vi "Initialize.vi"(8 "error in (no error)":errorcluster, 9 "Reset (True)":bool=TRUE, 10 "ID Query (True)":bool=TRUE, 11 "VISA resource name":refnum<visa-resource-name>) -> (0 "error out":errorcluster, 3 "VISA resource name out":refnum<visa-resource-name>)   [LabVIEW 2016, in "Keithley DMM6500 DAQ6500 Series.lvlib"]
doc: "Establishes communication with the instrument and optionally performs an instrument identification query and/or an instrument reset. It also places the instrument in a default state needed for other instrument driver operations. Therefore, call this VI before calling other instrument driver VIs for this instrument. Generally, you need to call the <b>Initialize</b> VI only once at the beginning of an application."
uses:
  Keithley DMM6500 DAQ6500 Series.lvlib
panel:
  # "(c) 2018 National Instruments.  ALL RIGHTS RESERVED."
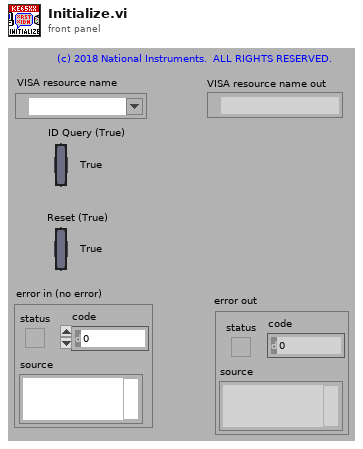
[diagram p1: front panel]
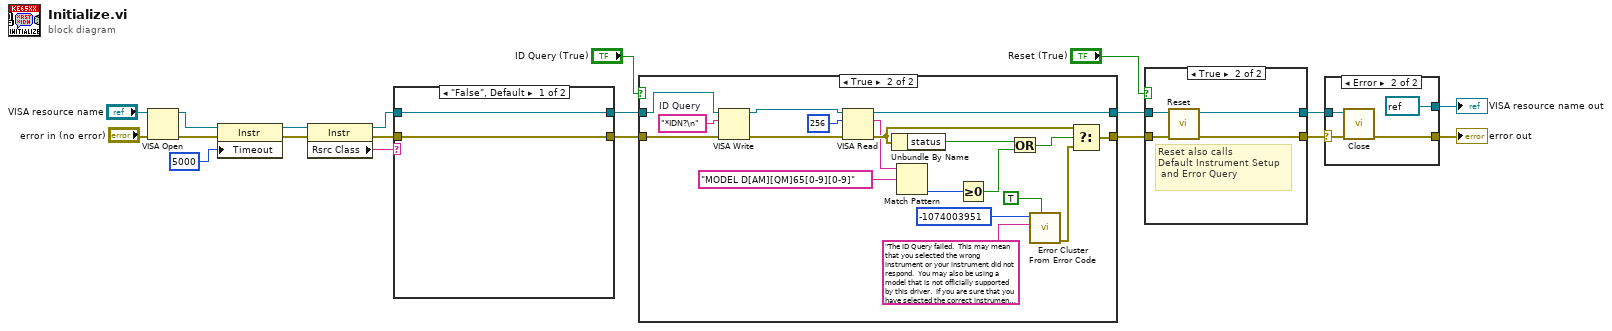
[diagram p0: block diagram]
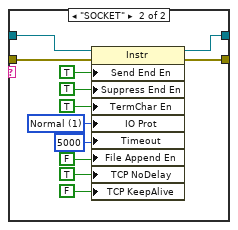
[diagram p2: hidden frame]
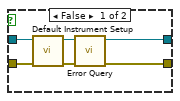
[diagram p4: hidden frame]
diagram:
  n1 = VISA Open(error in (no error)="error in (no error)", VISA resource name="VISA resource name") -> (VISA resource name=w4:refnum<visa-resource-name>, error out=w3:errorcluster)  [unwired: 3 in]
  n2 = property class="Instr"(reference=w4, error in=w3, "Timeout"=u32 5000 ("General Settings:Timeout Value")) -> (reference out=w1:refnum<visa-resource-name>, error out=w2:errorcluster)
  n3 = property class="Instr"(reference=w1, error in=w2) -> (reference out=w9:refnum<visa-resource-name>, error out=w8:errorcluster, "Rsrc Class"=w10:string)
  n4 = case shown="\"False\", Default" w10 {
    tunnel: w9 -> [w22 w31]
    tunnel: w8 -> [w21 w30]
    tunnel: [w22 w33] -> w7
    tunnel: [w21 w32] -> w6
    frame "False", Default {
    }
    frame "SOCKET" {
      w26 = u16 1 items=["Normal"=1, "VXI/FDC"=2, "GPIB/HS488"=3, "Serial-TCPIP-USB/488 Strings"=4, "USBTMC/Vendor-Specific"=5] ("Message Based Settings:IO Protocol")
      n5 = property class="Instr"(reference=w31, error in=w30, "Send End En"=TRUE ("Message Based Settings:Termination Character Enable"), "Suppress End En"=TRUE ("Message Based Settings:Suppress End Enable"), "TermChar En"=TRUE ("Message Based Settings:Termination Character Enable"), "IO Prot"=w26, "Timeout"=u32 5000 ("General Settings:Timeout Value"), "File Append En"=FALSE ("Message Based Settings:File Append Enable"), "TCP NoDelay"=TRUE ("TCP/IP Settings:No Packet Delay"), "TCP KeepAlive"=FALSE ("TCP/IP Settings:Keep-Alive Packets")) -> (reference out=w33:refnum<visa-resource-name>, error out=w32:errorcluster)
    }
  }
  n6 = case shown="True" "ID Query (True)" {
    tunnel: [w35 w55] -> w19
    tunnel: [w36 w54] -> w20
    tunnel: w7 -> [w36 w38]
    tunnel: w6 -> [w35 w37]
    frame False {
    }
    frame True {
      w49 = "*IDN?\n"  # ID Query
      n7 = VISA Write(VISA resource name=w38, write buffer=w49, error in (no error)=w37) -> (VISA resource name out=w53:refnum<visa-resource-name>, error out=w52:errorcluster)  [unwired: 1 out]
      n8 = VISA Read(VISA resource name=w53, byte count=u32 256, error in (no error)=w52) -> (VISA resource name out=w54:refnum<visa-resource-name>, read buffer=w39:string, error out=w43:errorcluster)  [unwired: 1 out]
      n9 = Unbundle By Name(w43) -> ("status"=w42:bool)
      n10 = Match Pattern(string=w39, regular expression="MODEL D[AM][QM]65[0-9][0-9]") -> (offset past match=w44:i32)  [unwired: 1 in, 3 out]
      n11 = Greater Or Equal To 0?(x=w44) -> (x >= 0?=w41:bool)
      n12 = Or(x=w42, y=w41) -> (x .or. y?=w40:bool)
      n13 = call <vilib>:"Error Cluster From Error Code.vi"("show call chain? (False)"=TRUE, "error message (\"\")"="The ID Query failed.  This may mean that you selected the wrong instrument or your instrument did not respond.  You may also be using a model that is not officially supported by this driver.  If you are sure that you have selected the correct instrument and it is responding, try disabling the ID Query." ("Source (VI Name)"), "error code (0)"=-1074003951 ("Code")) -> ("error out"=w48:errorcluster)  [unwired: 6 in]
      n14 = Select(t=w43, s=w40, f=w48) -> (s? t:f=w55:errorcluster)
    }
  }
  n15 = case shown="True" "Reset (True)" {
    tunnel: w19 -> [w60 w62]
    tunnel: [w57 w65] -> w11
    tunnel: w20 -> [w61 w63]
    tunnel: [w58 w64] -> w12
    frame False {
      n16 = call "Default Instrument Setup.vi"("error in (no error)"=w60, "VISA resource name"=w61) -> ("error out"=w56:errorcluster, "VISA resource name out"=w59:refnum<visa-resource-name>)  [unwired: 8 in]
      n17 = call "Error Query.vi"("error in (no error)"=w56, "VISA resource name"=w59) -> ("error out"=w57:errorcluster, "VISA resource name out"=w58:refnum<visa-resource-name>)  [unwired: 6 in, 2 out]
    }
    frame True {
      # "Reset also calls \nDefault Instrument Setup\n and Error Query"
      n18 = call "Reset.vi"("error in (no error)"=w62, "VISA resource name"=w63) -> ("error out"=w65:errorcluster, "VISA resource name out"=w64:refnum<visa-resource-name>)  [unwired: 8 in]
    }
  }
  n19 = case shown="Error" w11 {
    selector: w11 -> [w66 w69]
    tunnel: w12 -> [w67 w70]
    tunnel: [w67 refnum<visa-resource-name> refnum ("VISA resource name out")] -> w14
    tunnel: [w66 w71] -> w13
    frame No Error {
    }
    frame Error {
      n20 = call "Close.vi"("error in (no error)"=w69, "VISA resource name"=w70) -> ("error out"=w71:errorcluster)  [unwired: 9 in]
    }
  }
  "VISA resource name out" <- w14
  "error out" <- w13
